vi "ActionVIOnLoad.vi"(8 "error in (no error)":errorcluster, 11 "Device Item Ref in":T1 format="%.0x") -> (0 "error out":errorcluster, 3 "Device Item Ref out":T1 format="%.0x")   [LabVIEW 2016, in "FPGA Addon System Explorer.lvlib"]
uses:
  FPGA Addon System Explorer.lvlib
  <vilib>/NI Veristand/Custom Device API/Custom Device Item Ref.ctl
  Shared/FG Action.ctl
  NationalInstruments.VeriStand.SystemDefinitionAPI
  <vilib>/NI Veristand/Custom Device API/Get Item Property (Path).vi
  <vilib>/NI Veristand/Custom Device API/Get Item Property (String).vi
  <vilib>/NI Veristand/Custom Device API/NI VeriStand - Set Item Property.vi
  <vilib>/NI Veristand/Custom Device API/Set Item Property (Path).vi
  <vilib>/NI Veristand/Custom Device API/Set Item Property (String).vi
  <vilib>/NI VeriStand/Custom Device API/Custom Device API.lvlib
  Shared/Constants.vi
  Shared/FPGA Addon Shared.lvlib
  <vilib>/NI VeriStand/Custom Device Tools/Custom Device Utility Library/Custom Device Utility Library.lvlib
  <vilib>/NI Veristand/Custom Device Tools/Custom Device Utility Library/NI VeriStand - Search for Item by GUID.vi
  Shared/Data Type.ctl
  Shared/Register Information.ctl
  <vilib>/NI Veristand/Custom Device API/Get Item Property (Variant).vi
  FPGA-Resource-Manager-APIs/Source/Shared/FPGA RM Shared API.lvlib
  FPGA-Resource-Manager-APIs/Source/System Definition/FPGA RM System Definition API.lvlib
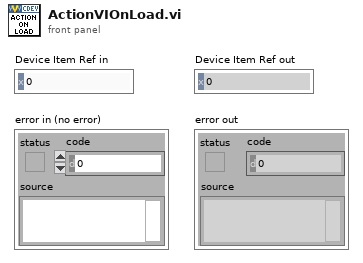
[diagram p1: front panel]
types:
  T1 = typedef "Custom Device API.lvlib/Custom Device Item Ref.ctl" = u64
  T2 = typedef "FPGA Addon Shared.lvlib/Register Information.ctl" = cluster{"Name":string, "Data Type":T3, "Default Value":variant}
  T3 = typedef "FPGA RM System Definition API.lvlib/Data Type.ctl" = enum8{"<Null>", "I8", "I16", "I32", "I64", "U8", "U16", "U32", "U64", "SGL", "Boolean", "Analog PWM In Settings", "Analog PWM In", "Digital PWM In Settings", "Digital PWM In", "Digital PWM Out", "Sine Out", "FXP+/-24.5", "FXP+/-16.5", "FXP+/-32.8", "FXP+/-64.32", "FXP+/-16.7", "FXP+/-20.5"}
  T4 = typedef "FPGA Addon Shared.lvlib/Data Type.ctl" = enum8{"<Null>", "I8", "I16", "I32", "I64", "U8", "U16", "U32", "U64", "SGL", "Boolean", "Analog PWM In Settings", "Analog PWM In", "Digital PWM In Settings", "Digital PWM In", "Digital PWM Out", "Sine Out", "FXP+/-24.5", "FXP+/-16.5", "FXP+/-32.8", "FXP+/-64.32", "FXP+/-16.7", "FXP+/-20.5"}
  T5 = typedef "FPGA RM Shared API.lvlib/FG Action.ctl" = enum8{"GET", "SET"}
  T6 = cluster{"Name":string, "Data Type":enum8{"<Null>", "I8", "I16", "I32", "I64", "U8", "U16", "U32", "U64", "SGL", "DBL", "EXT", "CSG", "CDB", "CXT", "0x0F", "0x10", "0x11", "0x12", "0x13", "0x14", "Enum U8", "Enum U16", "Enum U32", "Enum U64", "SGL PQ", "DBL PQ", "EXT PQ", "CSG PQ", "CDB PQ", "CXT PQ", "0x1F", "0x20", "Boolean", "0x22", "0x23", "0x24", "0x25", "0x26", "0x27", "0x28", "0x29", "0x2A", "0x2B", "0x2C", "0x2D", "0x2E", "0x2F", "String", "0x31", "Path", "Pict", "0x34", "0x35", "0x36", "DAQ", "0x38", "0x39", "0x3A", "0x3B", "0x3C", "0x3D", "0x3E", "0x3F", "Array", "0x41", "0x42", "0x43", "0x44", "0x45", "0x46", "0x47", "0x48", "0x49", "0x4A", "0x4B", "0x4C", "0x4D", "0x4E", "0x4F", "Cluster", "0x51", "0x52", "Variant", "Waveform", "0x55", "0x56", "0x57", "0x58", "0x59", "0x5A", "0x5B", "0x5C", "0x5D", "0x5E", "0x5F", "0x60", "0x61", "0x62", "0x63", "0x64", "0x65", "0x66", "0x67", "0x68", "0x69", "0x6A", "0x6B", "0x6C", "0x6D", "0x6E", "0x6F", "Refnum"}, "Default Value":dbl}[]
  T7 = enum8{"<Null>", "I8", "I16", "I32", "I64", "U8", "U16", "U32", "U64", "SGL", "DBL", "EXT", "CSG", "CDB", "CXT", "0x0F", "0x10", "0x11", "0x12", "0x13", "0x14", "Enum U8", "Enum U16", "Enum U32", "Enum U64", "SGL PQ", "DBL PQ", "EXT PQ", "CSG PQ", "CDB PQ", "CXT PQ", "0x1F", "0x20", "Boolean", "0x22", "0x23", "0x24", "0x25", "0x26", "0x27", "0x28", "0x29", "0x2A", "0x2B", "0x2C", "0x2D", "0x2E", "0x2F", "String", "0x31", "Path", "Pict", "0x34", "0x35", "0x36", "DAQ", "0x38", "0x39", "0x3A", "0x3B", "0x3C", "0x3D", "0x3E", "0x3F", "Array", "0x41", "0x42", "0x43", "0x44", "0x45", "0x46", "0x47", "0x48", "0x49", "0x4A", "0x4B", "0x4C", "0x4D", "0x4E", "0x4F", "Cluster", "0x51", "0x52", "Variant", "Waveform", "0x55", "0x56", "0x57", "0x58", "0x59", "0x5A", "0x5B", "0x5C", "0x5D", "0x5E", "0x5F", "0x60", "0x61", "0x62", "0x63", "0x64", "0x65", "0x66", "0x67", "0x68", "0x69", "0x6A", "0x6B", "0x6C", "0x6D", "0x6E", "0x6F", "Refnum"}
  T8 = typedef "FPGA Addon Shared.lvlib/FPGA Settings.ctl" = cluster{"Bitfile path":path, "RIO Device Address":string}
  T9 = typedef "Custom Device API.lvlib/Custom Device Item Info.ctl" = cluster{"Name":string, "Is Channel":bool, "GUID":string, "Is Waveform":bool}
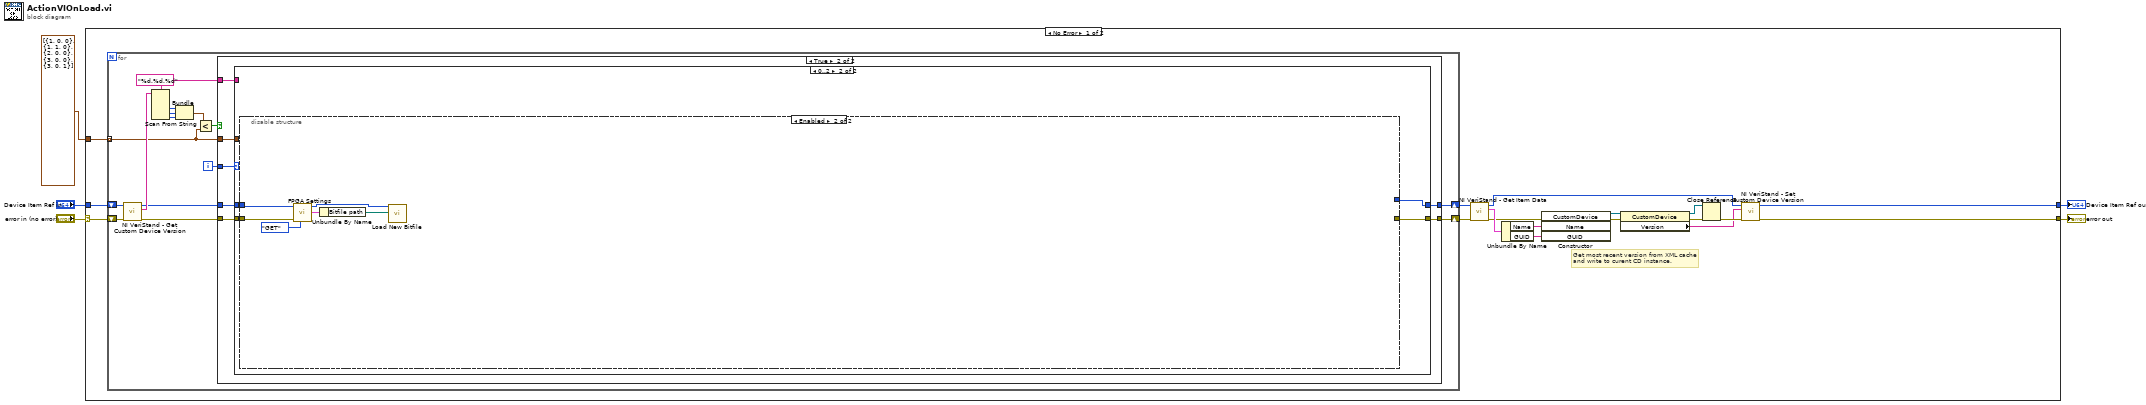
[diagram p0: block diagram]
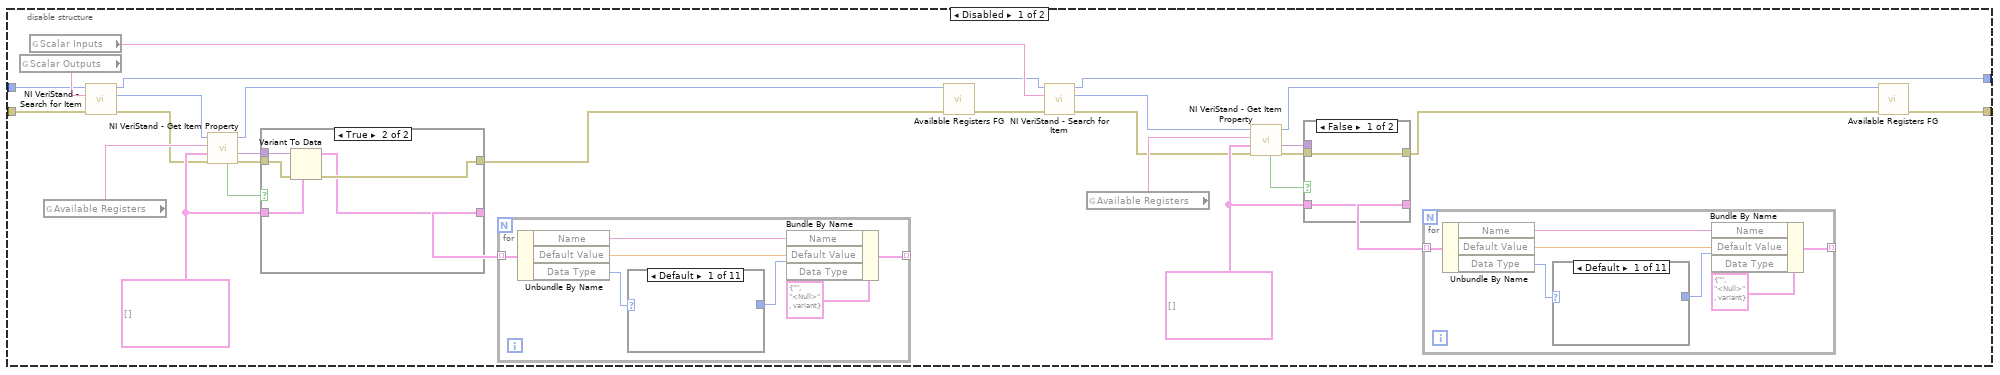
[diagram p4: hidden frame]
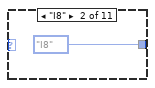
[diagram p5: hidden frame]
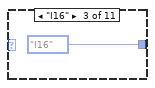
[diagram p6: hidden frame]
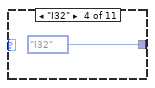
[diagram p7: hidden frame]
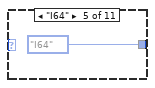
[diagram p8: hidden frame]
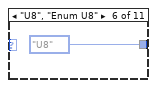
[diagram p9: hidden frame]
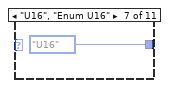
[diagram p10: hidden frame]
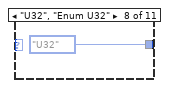
[diagram p11: hidden frame]
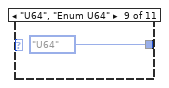
[diagram p12: hidden frame]
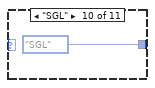
[diagram p13: hidden frame]
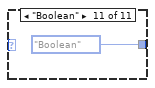
[diagram p14: hidden frame]
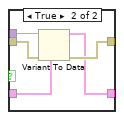
[diagram p15: hidden frame]
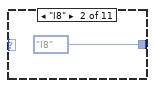
[diagram p16: hidden frame]
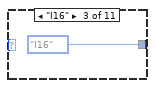
[diagram p17: hidden frame]
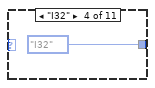
[diagram p18: hidden frame]
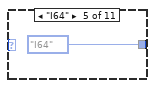
[diagram p19: hidden frame]
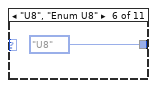
[diagram p20: hidden frame]
diagram:
  n1 = case shown="No Error" "error in (no error)" {
    selector: "error in (no error)" -> [w22 w137]
    tunnel: [w8 w137] -> w2
    tunnel: "Device Item Ref in" -> [w21 w136]
    tunnel: [w6 w136] -> w1
    tunnel: cluster{i32, i32, i32}[] [{1, 0, 0}, {1, 1, 0}, {2, 0, 0}, {3, 0, 0}, {3, 0, 1}] -> [w23 _]
    frame No Error {
      # "Get most recent version from XML cache\nand write to curent CD instance."
      n2 = for {
        tunnel: w23 -> [w26] mode=indexing
        shift-right: [w31] -> w9
        shift-left: w22 -> [w36]
        shift-right: [w29] -> w7
        shift-left: w21 -> [w35]
        i -> [w28]
        w27 = "%d.%d.%d" ("format string")
        n3 = call <vilib>:"NI VeriStand - Get Custom Device Version.vi"("error in (no error)"=w36, "Device Ref in"=w35) -> ("error out"=w32:errorcluster, "Value"=w34:string, "Device Ref out"=w30:T1)  [unwired: 7 in]
        n4 = Scan From String(format string=w27, input string=w34) -> (output 1=w37:i32, output 2=w38:i32, output 3=w25:i32)  [unwired: 5 in, 3 out]
        n5 = Bundle(w37, w38, w25) -> (w24:cluster{i32, i32, i32})  [unwired: 1 in]
        n6 = Less?(x=w24, y=w26) -> (x < y?=w33:bool)
        n7 = case shown="True" w33 {
          tunnel: w32 -> [w40 w47]
          tunnel: [w40 w46] -> w31
          tunnel: w30 -> [w39 w43]
          tunnel: [w39 w44] -> w29
          tunnel: w28 -> [_ w45]
          tunnel: w26 -> [_ w42]
          tunnel: w27 -> [_ w41]
          frame False {
          }
          frame True {
            n8 = case shown="0..2" w45 {
              tunnel: w47 -> [w49 w53]
              tunnel: [w49 w50] -> w46
              tunnel: [w48 w51] -> w44
              tunnel: w43 -> [w48 w52]
              tunnel: w42 -> [_ _]
              tunnel: w41 -> [_ _]
              frame Default {
              }
              frame 0..2 {
                n9 = disable-structure shown="Enabled" {
                  disable-tunnel: w53 -> [w78 w134]
                  disable-tunnel: w52 -> [w77 w135]
                  disable-tunnel: [w56 _] -> w51
                  disable-tunnel: [w55 _] -> w50
                  frame Disabled {
                    w62 = T6 [] ("Available Registers 2")
                    w72 = T6 [] ("Available Registers 2")
                    n10 = global read "Constants.vi" "Scalar Outputs"() -> (w81:string)
                    n11 = global read "Constants.vi" "Scalar Inputs"() -> (w79:string)
                    n12 = global read "Constants.vi" "Available Registers"() -> (w73:string)
                    n13 = call-poly <vilib>:"NI VeriStand - Search for Item.vi"("error in"=w78, "Item GUID"=w81, "Section Ref in"=w77) -> ("error out"=w69:errorcluster, "Item Ref"=w71:T1, "Section Ref out"=w54:T1)  [unwired: 5 in, 1 out]
                    n14 = call-poly <vilib>:"NI VeriStand - Get Item Property.vi"("error in (no error)"=w69, "Default Value"=w72, "Property Name"=w73, "Item Ref in"=w71) -> ("error out"=w75:errorcluster, "Value"=w74:variant, "Item Ref out"=w70:T1, "Found?"=w76:bool)  [unwired: 4 in]
                    n15 = case shown="True" w76 {
                      tunnel: w74 -> [_ w129]
                      tunnel: w72 -> [w123 w128]
                      tunnel: w75 -> [w124 w127]
                      tunnel: [w124 w126] -> w68
                      tunnel: [w123 w125] -> w67
                      frame False {
                      }
                      frame True {
                        n16 = Variant To Data(error in=w127, type=w128, Variant=w129) -> (data=w125:T6, error out=w126:errorcluster)
                      }
                    }
                    n17 = for {
                      tunnel: w67 -> [w112] mode=indexing
                      tunnel: [w108] -> _ mode=indexing
                      n18 = Unbundle By Name(w112) -> ("Name"=w111:string, "Default Value"=w110:dbl, "Data Type"=w107:T7)
                      n19 = case shown="Default" w107 {
                        tunnel: [_ Data_Type."I8" ("Data Type") Data_Type."I16" ("Data Type") Data_Type."I32" ("Data Type") Data_Type."I64" ("Data Type") Data_Type."U8" ("Data Type") Data_Type."U16" ("Data Type") Data_Type."U32" ("Data Type") Data_Type."U64" ("Data Type") Data_Type."SGL" ("Data Type") Data_Type."Boolean" ("Data Type")] -> w106
                        frame Default {
                        }
                        frame "I8" {
                        }
                        frame "I16" {
                        }
                        frame "I32" {
                        }
                        frame "I64" {
                        }
                        frame "U8", "Enum U8" {
                        }
                        frame "U16", "Enum U16" {
                        }
                        frame "U32", "Enum U32" {
                        }
                        frame "U64", "Enum U64" {
                        }
                        frame "SGL" {
                        }
                        frame "Boolean" {
                        }
                      }
                      n20 = Bundle By Name(cluster=T2 {"Name"="", "Data Type"=enum."<Null>", "Default Value"=variant(refnum<class> refnum)}, "Name"=w111, "Default Value"=w110, "Data Type"=w106) -> (w108:T2)
                    }
                    n21 = call "Available Registers FG.vi"("error in (no error)"=w68, "Item Ref"=w70) -> ("error out"=w80:errorcluster)  [unwired: 7 in, 2 out]
                    n22 = call-poly <vilib>:"NI VeriStand - Search for Item.vi"("error in"=w80, "Item GUID"=w79, "Section Ref in"=w54) -> ("error out"=w60:errorcluster, "Item Ref"=w58:T1, "Section Ref out"=w56:T1)  [unwired: 5 in, 1 out]
                    n23 = global read "Constants.vi" "Available Registers"() -> (w63:string)
                    n24 = call-poly <vilib>:"NI VeriStand - Get Item Property.vi"("error in (no error)"=w60, "Default Value"=w62, "Property Name"=w63, "Item Ref in"=w58) -> ("error out"=w65:errorcluster, "Value"=w64:variant, "Item Ref out"=w57:T1, "Found?"=w66:bool)  [unwired: 4 in]
                    n25 = case shown="False" w66 {
                      tunnel: w64 -> [_ w105]
                      tunnel: w62 -> [w99 w104]
                      tunnel: w65 -> [w100 w103]
                      tunnel: [w100 w102] -> w59
                      tunnel: [w99 w101] -> w61
                      frame False {
                      }
                      frame True {
                        n26 = Variant To Data(error in=w103, type=w104, Variant=w105) -> (data=w101:T6, error out=w102:errorcluster)
                      }
                    }
                    n27 = for {
                      tunnel: w61 -> [w88] mode=indexing
                      tunnel: [w84] -> _ mode=indexing
                      n28 = Unbundle By Name(w88) -> ("Name"=w87:string, "Default Value"=w86:dbl, "Data Type"=w83:T7)
                      n29 = case shown="Default" w83 {
                        tunnel: [_ Data_Type."I8" ("Data Type") Data_Type."I16" ("Data Type") Data_Type."I32" ("Data Type") Data_Type."I64" ("Data Type") Data_Type."U8" ("Data Type") Data_Type."U16" ("Data Type") Data_Type."U32" ("Data Type") Data_Type."U64" ("Data Type") Data_Type."SGL" ("Data Type") Data_Type."Boolean" ("Data Type")] -> w82
                        frame Default {
                        }
                        frame "I8" {
                        }
                        frame "I16" {
                        }
                        frame "I32" {
                        }
                        frame "I64" {
                        }
                        frame "U8", "Enum U8" {
                        }
                        frame "U16", "Enum U16" {
                        }
                        frame "U32", "Enum U32" {
                        }
                        frame "U64", "Enum U64" {
                        }
                        frame "SGL" {
                        }
                        frame "Boolean" {
                        }
                      }
                      n30 = Bundle By Name(cluster=T2 {"Name"="", "Data Type"=enum."<Null>", "Default Value"=variant(refnum<class> refnum)}, "Name"=w87, "Default Value"=w86, "Data Type"=w82) -> (w84:T2)
                    }
                    n31 = call "Available Registers FG.vi"("error in (no error)"=w59, "Item Ref"=w57) -> ("error out"=w55:errorcluster)  [unwired: 7 in, 2 out]
                  }
                  frame Enabled {
                    n32 = call "FPGA Settings.vi"("Action"=FG_Action."GET", "error in (no error)"=w134, "Item Ref"=w135) -> ("FPGA Settings"=w132:T8, "Item Ref out"=w130:T1)  [unwired: 6 in, 1 out]
                    n33 = Unbundle By Name(w132) -> ("Bitfile path"=w131:path)
                    n34 = call "Load New Bitfile.vi"("NewVal"=w131, "Item Ref in"=w130) -> ()  [unwired: 8 in, 2 out]
                  }
                }
              }
            }
          }
        }
      }
      n35 = call <vilib>:"NI VeriStand - Get Item Data.vi"("error in (no error)"=w9, "Item Ref in"=w7) -> ("error out"=w17:errorcluster, "Item Info"=w20:T9, "Item Ref out"=w10:T1)  [unwired: 6 in, 1 out]
      n36 = Unbundle By Name(w20) -> ("Name"=w19:string, "GUID"=w18:string)
      n37 = constructor class="CustomDevice"(error in=w17, "Name"=w19, "GUID"=w18) -> (reference out=w16:refnum<k24>, error out=w15:errorcluster)  [unwired: 2 in, 3 out]
      n38 = property class="CustomDevice"(reference=w16, error in=w15) -> (reference out=w13:refnum<k24>, error out=w14:errorcluster, "Version"=w11:string)
      n39 = Close Reference(reference=w13, error in (no error)=w14) -> (error out=w12:errorcluster)
      n40 = call <vilib>:"NI VeriStand - Set Custom Device Version.vi"("error in (no error)"=w12, "Value"=w11, "Device Ref in"=w10) -> ("error out"=w8:errorcluster, "Device Ref out"=w6:T1)  [unwired: 7 in]
    }
    frame Error {
    }
  }
  "error out" <- w2
  "Device Item Ref out" <- w1
